vi "add transfer to configuration.vi"(8 "error in (no error)":errorcluster, 9 "transfer info":T1, 10 "id":string, 11 "DSFConfiguration in":refnum<class "DSFConfiguration.lvclass">) -> (0 "error out":errorcluster, 3 "DSFConfiguration out":refnum<class "DSFConfiguration.lvclass">)   [LabVIEW 2017, in "DSFConfiguration.lvclass"]
uses:
  DSFConfiguration.lvclass
  IDable/IDable.lvclass
  DSFTransfer/DSFTransfer.lvclass
  C:/github/data-sharing-framework-custom-device/Source/Submodules/DSF/Source/Configuration API/Classes/IDable/IDable.lvclass
  Controls/dsf configuration file/1.0.0/dsf transfer.ctl
  Controls/dsf configuration file/1.0.0/dsf configuration file v1.0.0.lvlib
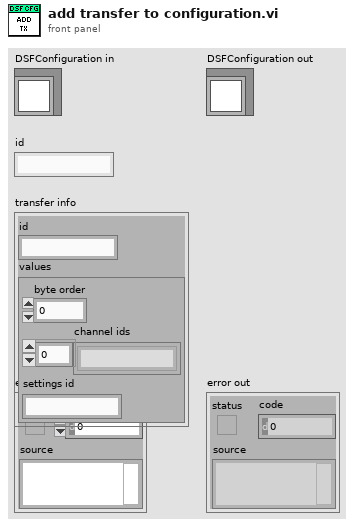
[diagram p1: front panel]
types:
  T1 = typedef "dsf configuration file v1.0.0.lvlib/dsf transfer.ctl" = cluster{"id":string, "values":cluster{"byte order":i32, "channel ids":string[], "settings id":string}}
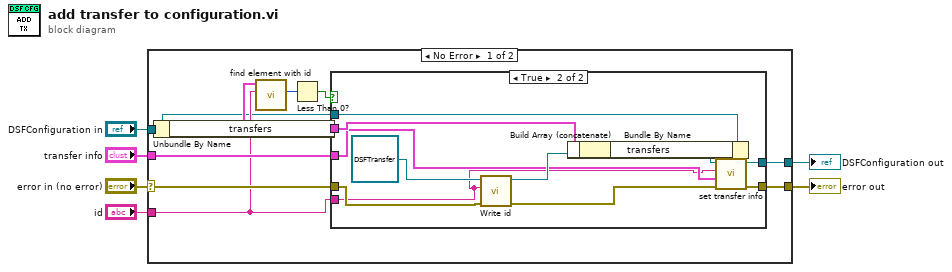
[diagram p0: block diagram]
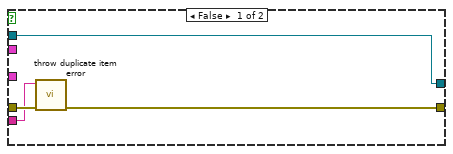
[diagram p2: hidden frame]
diagram:
  n1 = case shown="No Error" "error in (no error)" {
    selector: "error in (no error)" -> [w11 w33]
    tunnel: [w12 w33] -> w1
    tunnel: "DSFConfiguration in" -> [w7 w32]
    tunnel: "id" -> [w9 _]
    tunnel: "transfer info" -> [w10 _]
    tunnel: [w8 w32] -> w2
    frame No Error {
      n2 = Unbundle By Name(w7) -> ("transfers"=w13:T1[])
      n3 = call "find element with id.vi"("id"=w9, "IDable Array in"=w13) -> ("index"=w15:i32)  [unwired: 8 in, 1 out]
      n4 = Less Than 0?(x=w15) -> (x < 0?=w14:bool)
      n5 = case shown="True" w14 {
        tunnel: w13 -> [_ w31]
        tunnel: [w18 w27] -> w12
        tunnel: w11 -> [w17 w21]
        tunnel: w10 -> [_ w22]
        tunnel: w9 -> [w16 w20]
        tunnel: w7 -> [w19 w25]
        tunnel: [w19 w26] -> w8
        frame False {
          n6 = call "throw duplicate item error.vi"("error in (no error)"=w17, "id"=w16) -> ("error out"=w18:errorcluster)  [unwired: 9 in]
        }
        frame True {
          n7 = call "Write id.vi"("error in (no error)"=w21, "id"=w20, "IDable in"=refnum<class "DSFTransfer.lvclass"> refnum ("DSFTransfer.lvclass")) -> ("error out"=w28:errorcluster, "IDable out"=w29:refnum<class "DSFTransfer.lvclass">)  [unwired: 7 in]
          n8 = Build Array (concatenate)(w31, w29) -> (w24:T1[])
          n9 = Bundle By Name(cluster=w25, "transfers"=w24) -> (w23:refnum<class "DSFConfiguration.lvclass">)
          n10 = call "set transfer info.vi"("error in (no error)"=w28, "transfer info"=w22, "id"=w20, "DSFConfiguration in"=w23) -> ("error out"=w27:errorcluster, "DSFConfiguration out"=w26:refnum<class "DSFConfiguration.lvclass">)  [unwired: 6 in]
        }
      }
    }
    frame Error {
    }
  }
  "error out" <- w1
  "DSFConfiguration out" <- w2
